vi "Returning A Value Array Of Integers Complete.vi"() -> ()   [LabVIEW 2009, in "LabVIEWWrapper_PassingDataSampleDLL.lvlib"]
uses:
  LabVIEWWrapper_PassingDataSampleDLL.lvlib
panel:
  out "error out":errorcluster
  in  "error in (no error)":errorcluster
  out "Value":i32[](array[numeric])
  in  "length":i32
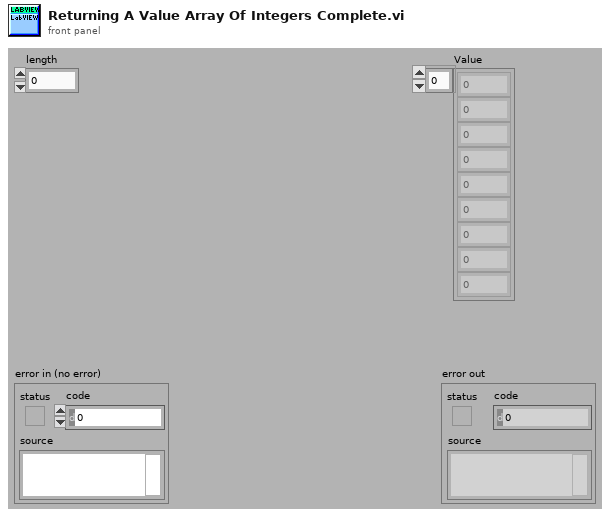
[diagram p1: front panel]
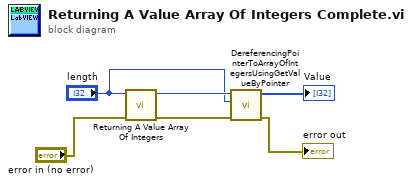
[diagram p0: block diagram]
diagram:
  n1 = call "Returning A Value Array Of Integers.vi"("error in (no error)"="error in (no error)", "length"="length") -> ("error out"=w1:errorcluster, "function return"=w3:i32)  [unwired: 8 in]
  n2 = call "DereferencingPointerToArrayOfIntegersUsingGetValueByPointer.vi"("error in (no error)"=w1, "Length"="length", "Address (Pointer)"=w3) -> ("error out"=→"error out":errorcluster, "Value"=→"Value":i32[])  [unwired: 7 in]
